vi "Close_Power_Meter.vi"(8 "error in (no error)":errorcluster, 11 "VISA resource name":refnum<visa-resource-name>="USB0::0x2A8D::0x1D01::MY55170004::INSTR") -> (0 "error out":errorcluster)   [LabVIEW 2015]
uses:
  <instrlib>/Agilent U2000 Series/Agilent U2000 Series.lvlib
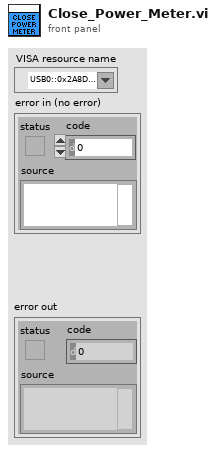
[diagram p1: front panel]
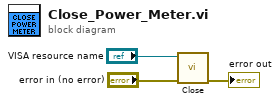
[diagram p0: block diagram]
diagram:
  n1 = call <instrlib>:"Close.vi"("error in (no error)"="error in (no error)", "VISA resource name"="VISA resource name") -> ("error out"=→"error out":errorcluster)  [unwired: 9 in]
